vi "target - single rate.vi"() -> ()   [LabVIEW 2020]
uses:
  <vilib>/RioEmbeddedCAN/RioEmbeddedCAN.llb/CANFrameControl.ctl
panel:
  out "Iteration":i32
  out "CAN input":T1
  out "CAN output":T2 {"type" items=["CAN Data", "CAN Remote"]; "identifier" format="%.0x"}
  in  "stop":bool
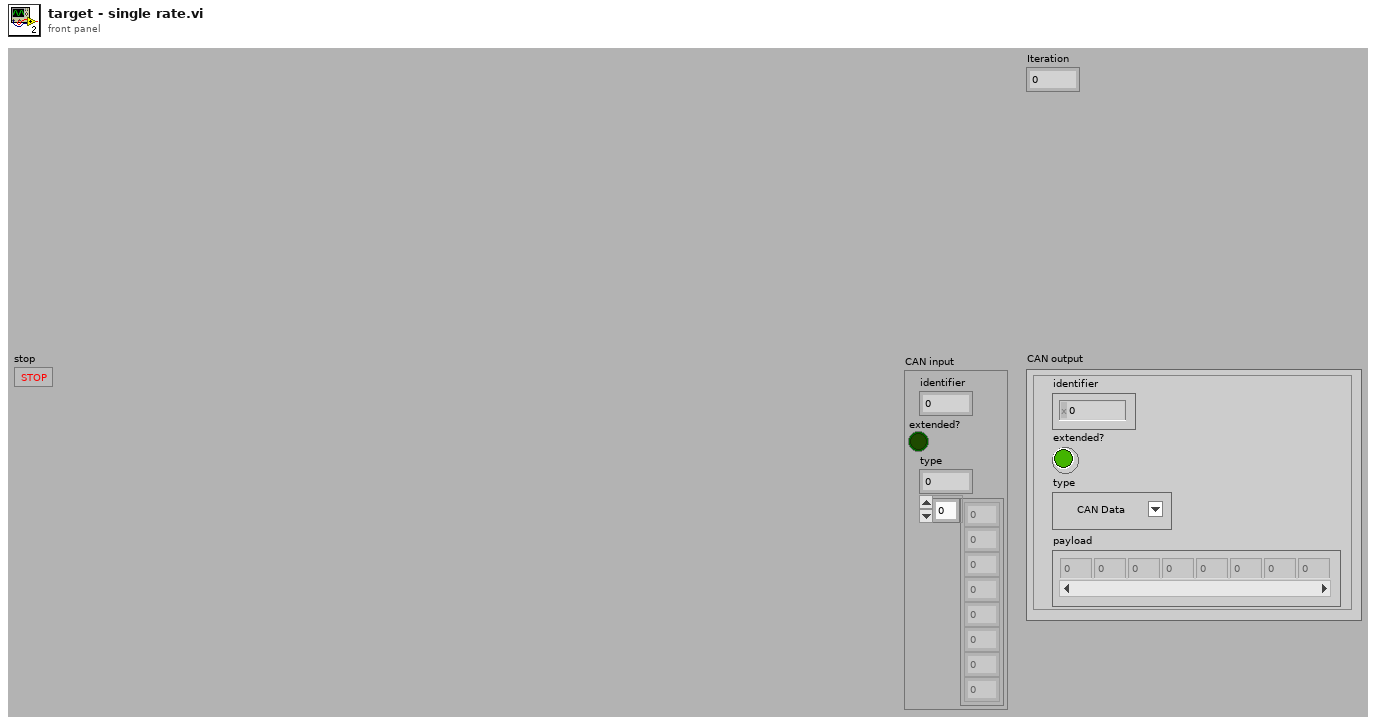
[diagram p1: front panel]
types:
  T1 = cluster{"identifier":u32, "extended?":bool, "type":u8, u64[]}
  T2 = typedef "CANFrameControl.ctl" = cluster{"identifier":u32, "extended?":bool, "type":u8, "payload":u8[]}
  T3 = cluster{"Weights (1000x2001)":dbl[][], "Weights (4x4x1000x15)":dbl[][][][], "Weights (4x4x15x8)":dbl[][][][], "Weights (4x9)":dbl[][]}
  T4 = cluster{"FPGA VI Reference Out":refnum<k20>, "error out":errorcluster}
  T5 = cluster{"Boolean":bool, "initialized array":string[][], "interface object out":refnum<k20>, "error out":errorcluster}
  T6 = cluster{"interface object out":refnum<k20>, "error out":errorcluster}
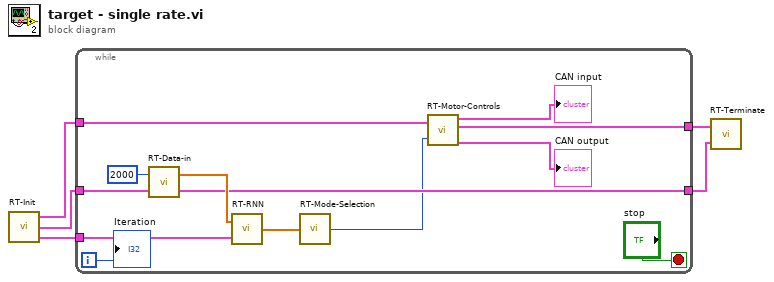
[diagram p0: block diagram]
diagram:
  n1 = call "RT-Init.vi"() -> ("Weights"=w3:T3, "Data-in Settings"=w5:T4, "Motor-Controller Settings"=w4:T5)
  n2 = while {
    tunnel: w5 -> [w14]
    tunnel: w4 -> [w13]
    tunnel: [w12] -> w1
    tunnel: [w11] -> w2
    tunnel: w3 -> [w8]
    i -> [w6]
    stop <- "stop" stop-if-true
    n3 = call "RT-Data-in.vi"("cluster"=w14, "Amount of Inputs"=2000) -> ("Error"=w11:T4, "Bicep+Triceps"=w18:dbl[])
    n4 = call "RT-RNN.vi"("Weights Cluster"=w8, "Input"=w18) -> ("Output"=w10:dbl[])
    n5 = call "RT-Mode-Selection.vi"("Array"=w10) -> ("U64-Output"=w9:u64)
    n6 = call "RT-Motor-Controls.vi"("Settings"=w13, "U64-Input"=w9) -> ("CAN input"=→"CAN input":T1, "Error"=w12:T6, "CAN output"=→"CAN output":T2)  [unwired: 1 in]
    "Iteration" <- w6
  }
  n7 = call "RT-Terminate.vi"("Data input"=w2, "Motor Controller"=w1) -> ()  [unwired: 1 in]
